vi "Modbus (SubVI).vi"(11 "Update rate":dbl) -> (1 "Off Hook":bool, 2 "Updating":bool, 3 "Communication Error":bool)   [LabVIEW 2018]
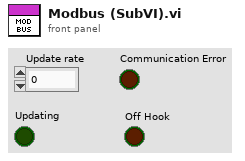
[diagram p1: front panel]
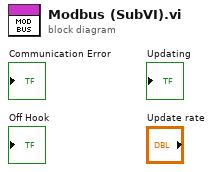
[diagram p0: block diagram]
diagram:
